vi "spk_voltage.vi"(7 "LVWSR":refnum<class "Web Request.lvclass">, 10 "Vscale":dbl, 11 "Voffset":dbl) -> ()   [LabVIEW 2016]
uses:
  <vilib>/wsapi/Web Request.lvclass
  Controller/Messages/Forward Command/Forward Command MSG.lvclass
  C:/Program Files (x86)/National Instruments/LabVIEW 2016/vi.lib/ActorFramework/Message/Message.lvclass
  PAS/Commands/Update Speaker Vscale Cmd/Update Speaker Vscale CMD.lvclass
  C:/Program Files (x86)/National Instruments/LabVIEW 2016/vi.lib/MSR Consulting, LLC/General Reuse/Command/Command.lvclass
  PAS/Commands/Update Speaker Vscale Cmd/Update Speaker Vscale CMD.lvclass/Update Speaker Vscale CMD.ctl
  Controller/Messages/Forward Command/Forward Command MSG.lvclass/Forward Command MSG.ctl
  <vilib>/ActorFramework/Message Enqueuer/Message Enqueuer.lvclass/Message Enqueuer.ctl
  PAS/Commands/Update Speaker Vscale Cmd/Write Voffset.vi
  PAS/Commands/Update Speaker Vscale Cmd/Write Vscale.vi
  Controller/Messages/Forward Command/Write id.vi
  Controller/Messages/Forward Command/Write CMD.vi
  <vilib>/ActorFramework/Message Priority Queue/Priority Enqueue.vi
  Controller/gController.lvclass
  <vilib>/ActorFramework/Message Enqueuer/Message Enqueuer.lvclass
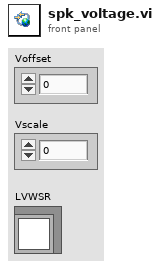
[diagram p1: front panel]
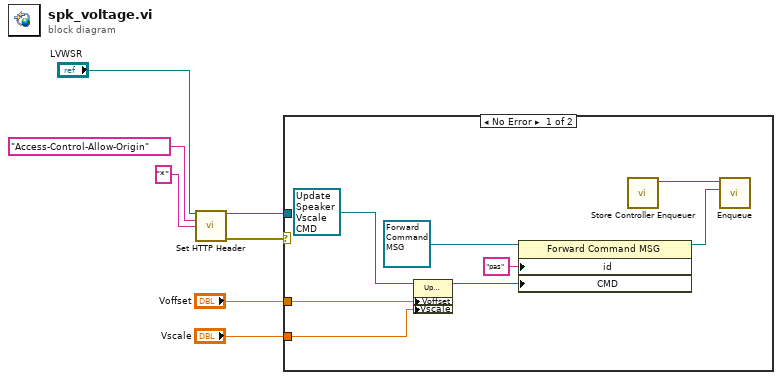
[diagram p0: block diagram]
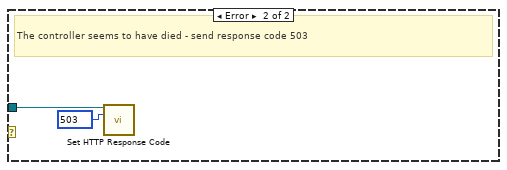
[diagram p2: hidden frame]
diagram:
  n1 = call <vilib>:"Set HTTP Header.vi"("LabVIEW Web Service Request"="LVWSR", "header"="Access-Control-Allow-Origin", "header value"="*") -> ("LabVIEW Web Service Request out"=w5:refnum<class "Web Request.lvclass">, "error out"=w4:errorcluster)  [unwired: 11 in]
  n2 = case shown="No Error" w4 {
    tunnel: w5 -> [_ w16]
    tunnel: "Voffset" -> [w9 _]
    tunnel: "Vscale" -> [w8 _]
    frame No Error {
      n3 = property class="Update Speaker Vscale CMD"(reference=refnum<class "Update Speaker Vscale CMD.lvclass"> refnum ("gPAS Library.lvlib:Update Speaker Vscale CMD"), "Voffset"=w9, "Vscale"=w8) -> (reference out=w11:refnum<class "Update Speaker Vscale CMD.lvclass">)  [unwired: 1 in, 1 out]
      n4 = property class="Forward Command MSG"(reference=refnum<class "Forward Command MSG.lvclass"> refnum ("Controller.lvlib:Forward Command MSG.lvclass"), "id"="pas", "CMD"=w11) -> (reference out=w13:refnum<class "Forward Command MSG.lvclass">)  [unwired: 1 in, 1 out]
      n5 = call "Store Controller Enqueuer.vi"() -> ("Controller Enqueuer Out"=w15:refnum<class "Message Enqueuer.lvclass">)  [unwired: 11 in]
      n6 = call <vilib>:"Enqueue.vi"("Message"=w13, "Message Enqueuer in"=w15) -> ()  [unwired: 8 in, 2 out]
    }
    frame Error {
      w17 = 503 items=["100"=100, "101"=101, "200"=200, "201"=201, "202"=202, "203"=203, "204"=204, "205"=205, "206"=206, "300"=300, "301"=301, "302"=302, "303"=303, "304"=304, "305"=305, "306"=306, "307"=307, "400"=400, "401"=401, "402"=402, "403"=403, "404"=404, "405"=405, "406"=406, "407"=407, "408"=408, "409"=409, "410"=410, "411"=411, "412"=412, "413"=413, "414"=414, "415"=415, "416"=416, "417"=417, "500"=500, "501"=501, "502"=502, "503"=503, "504"=504, "505"=505] ("response code (200)")
      # "The controller seems to have died - send response code 503"
      n7 = call <vilib>:"Set HTTP Response Code.vi"("LabVIEW Web Service Request"=w16, "response code (200)"=w17) -> ()  [unwired: 12 in, 2 out]
    }
  }
